vi "Filtro_EMA_Base.vi"() -> ()   [LabVIEW 2020]
panel:
  out "appended array":dbl[](array[numeric])
  out "Numeric 2":dbl
  in  "Array 2":dbl[](array[numeric])
  in  "stop":bool
  out "Array 3":dbl[](array[numeric])
  out "Numeric":dbl
  in  "Array":dbl[](array[numeric])
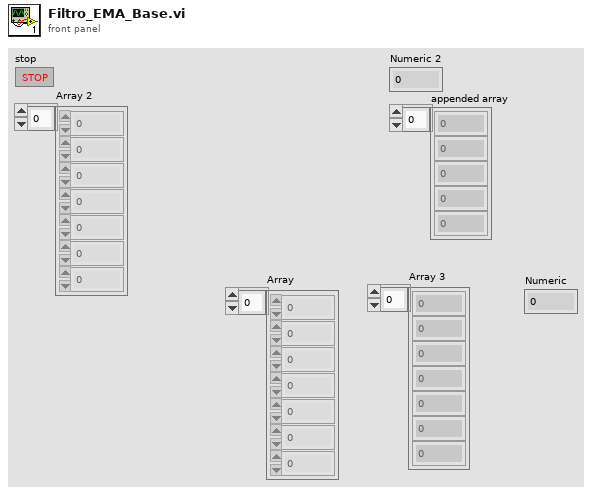
[diagram p1: front panel]
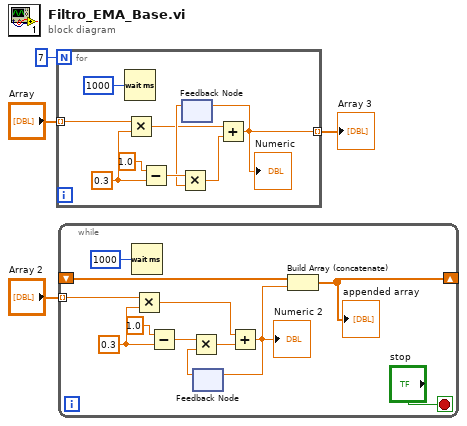
[diagram p0: block diagram]
diagram:
  n1 = for {
    N: 7 -> [_]
    tunnel: "Array" -> [w13] mode=indexing
    tunnel: [w5] -> w3 mode=indexing
    w11 = 0.3 ("y")
    n2 = Wait (ms)(milliseconds to wait=u32 1000) -> ()  [unwired: 1 out]
    n3 = Multiply(x=w13, y=w11) -> (x*y=w7:dbl)
    n4 = Subtract(x=1.0, y=w11) -> (x-y=w10:dbl)
    n5 = feedback #1() -> (w9:dbl)  [unwired: 1 in]
    n6 = Multiply(x=w10, y=w9) -> (x*y=w8:dbl)
    n7 = Add(x=w7, y=w8) -> (x+y=w5:dbl)
    "Numeric" <- w5
    n8 = feedback-in #1(w5) -> ()
  }
  "Array 3" <- w3
  n9 = while {
    tunnel: "Array 2" -> [w17] mode=indexing
    shift-right: [w15] -> _
    shift-left: _ -> [w14]
    stop <- "stop" stop-if-true
    w19 = 0.3 ("y")
    n10 = Wait (ms)(milliseconds to wait=u32 1000) -> ()  [unwired: 1 out]
    n11 = Multiply(x=w17, y=w19) -> (x*y=w23:dbl)
    n12 = Subtract(x=1.0, y=w19) -> (x-y=w20:dbl)
    n13 = feedback #2() -> (w21:dbl)  [unwired: 1 in]
    n14 = Multiply(x=w20, y=w21) -> (x*y=w22:dbl)
    n15 = Add(x=w23, y=w22) -> (x+y=w16:dbl)
    "Numeric 2" <- w16
    n16 = feedback-in #2(w16) -> ()
    n17 = Build Array (concatenate) "Build Array"(w14, w16) -> (w15:dbl[])
    "appended array" <- w15
  }
